vi "Test Process Stop without Start.vi"(8 "error in (no error)":errorcluster, 11 "Process Test In":refnum<class "Process Test.lvclass">) -> (0 "error out":errorcluster, 3 "Process Test Out":refnum<class "Process Test.lvclass">)   [LabVIEW 2020, in "Process Test.lvclass"]
uses:
  Process Test.lvclass
  C:/Users/anton/Documents/GitHub/Triarc-Framework/source/Framework Test/Base Class Test/Base Test.lvclass
  C:/Program Files (x86)/National Instruments/LabVIEW 2020/vi.lib/Asteme/LUnit/Test Case.lvclass
  Framework/Process/Process.lvclass
  Base Class Test/Base Test.lvclass/Base Test.ctl
  Framework/Process/Process.lvclass/Process.ctl
  <vilib>/Asteme/LUnit/Test Case.lvclass/Test Case.ctl
  <vilib>/Asteme/LUnit/LUnit Assertion Result.lvclass/LUnit Assertion Result.ctl
  Framework/Process/Public/Lifecycle/Get Lifecycle State.vi
  Framework/Process/Private/SubVIs/Wait for finish.vi
  Framework/Process/Protected/Messaging/Enqueue Message.vi
  Framework/Process/Private/SubVIs/Set Lifecycle State.vi
  <vilib>/Asteme/LUnit/Palette/Fail.vi
  <vilib>/Asteme/LUnit/Palette/Pass.vi
  <vilib>/Asteme/LUnit/Set Assertion Type.vi
  <vilib>/Utility/error.llb/Clear Errors.vi
  <vilib>/Asteme/LUnit/Add test result.vi
  <vilib>/Asteme/LUnit/LUnit Write Passed.vi
  <vilib>/Asteme/LUnit/LUnit Get Test Case.vi
  <vilib>/Asteme/LUnit/Assertion Result/LUnit Get Test Name.vi
  <vilib>/Asteme/LUnit/LUnit Write Message.vi
  <vilib>/Asteme/LUnit/LUnit Write Description.vi
  <vilib>/Asteme/LUnit/LUnit Write Assertion Type.vi
  <vilib>/Asteme/LUnit/Read Test Case Name.vi
  <vilib>/Utility/error.llb/Error Cluster From Error Code.vi
  Framework/Base/Base.lvclass
  <vilib>/Asteme/LUnit/LUnit Assertion Result.lvclass
  <vilib>/Asteme/LUnit/Test Case.lvclass
  Base Class Test/Base Test.lvclass
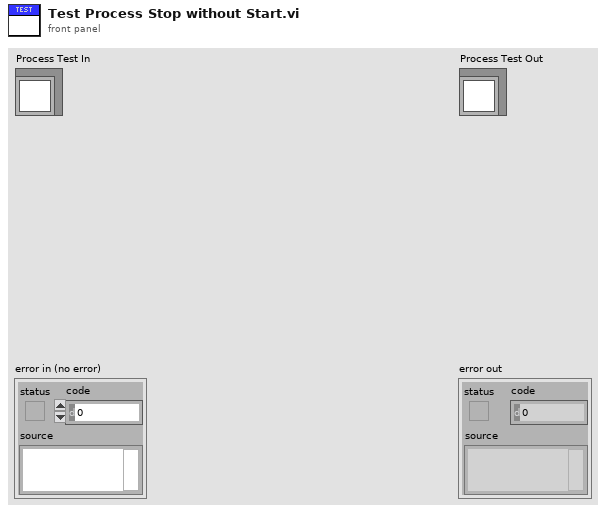
[diagram p1: front panel]
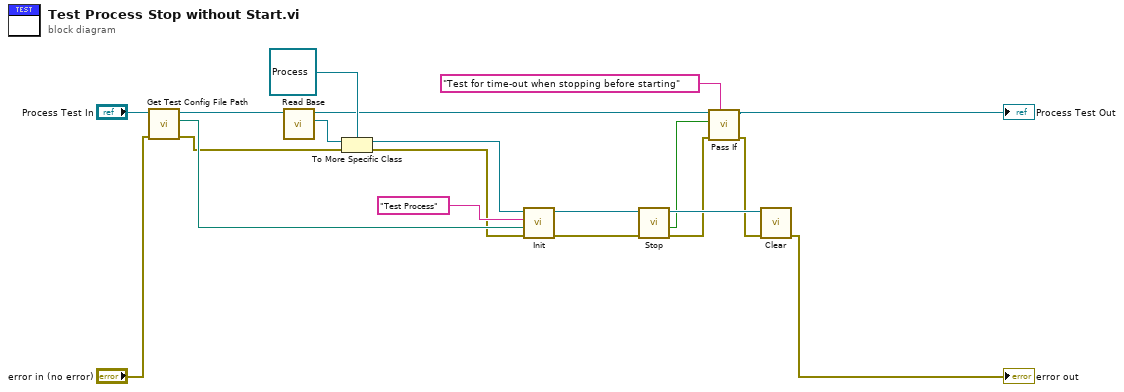
[diagram p0: block diagram]
diagram:
  n1 = call-dynamic "Get Test Config File Path.vi"("error in (no error)"="error in (no error)", "Base Class Test in"="Process Test In") -> ("error out"=w4:errorcluster, "Test config path"=w9:path, "Base Class Test out"=w6:refnum<class "Process Test.lvclass">)  [unwired: 7 in]
  n2 = call "Read Base.vi"("Base Class Test In"=w6) -> ("Base.lvclass"=w7:refnum<class "Base.lvclass">, "Base Class Test Out"=w5:refnum<class "Process Test.lvclass">)  [unwired: 8 in, 1 out]
  n3 = To More Specific Class(target class=refnum<class "Process.lvclass"> refnum ("Process.lvclass"), reference=w7, error in=w4) -> (specific class reference=w2:refnum<class "Process.lvclass">, error out=w3:errorcluster)
  n4 = call-dynamic "Init.vi"("error in (no error)"=w3, "Config File Path"=w9, "Name"="Test Process", "Process In"=w2) -> ("error out"=w12:errorcluster, "Process Out"=w15:refnum<class "Process.lvclass">)  [unwired: 6 in]
  n5 = call "Stop.vi"("error in (no error)"=w12, "Process In"=w15) -> ("error out"=w18:errorcluster, "timed out?"=w19:bool, "Process Out"=w20:refnum<class "Process.lvclass">)  [unwired: 7 in]
  n6 = call <vilib>:"Pass If.vi"("Description"="Test for time-out when stopping before starting" ("custom report message (\"\")"), "error in (no error)"=w18, "Pass?"=w19, "Test Case In"=w5) -> ("error out"=w14:errorcluster, "Test Case Out"=→"Process Test Out":refnum<class "Process Test.lvclass">)  [unwired: 6 in]
  n7 = call-dynamic "Clear.vi"("error in (no error)"=w14, "Process In"=w20) -> ("error out"=→"error out":errorcluster)  [unwired: 8 in, 1 out]
